vi "MecaDrivePoseEst2_ResetPosition.vi"(6 "Pose":T7={"TRANSLATION"={"X"=0.0, "Y"=0.0}, "ROTATION"={"VALUE"=0.0, "COS"=1.0, "SIN"=0.0}} {"ROTATION"."SIN" format="%13.4f"; "ROTATION"."COS" format="%13.4f"; "ROTATION"."VALUE" format="%13.4f"; "TRANSLATION"."Y" format="%14.3f"; "TRANSLATION"."X" format="%14.3f"}, 9 "Module Positions":T1 {"RearRight" format="%19.3f"; "RearLeft" format="%19.3f"; "FrontRight" format="%19.3f"; "FrontLeft" format="%19.3f"}, 10 "Gyro":T2={"VALUE"=0.0, "COS"=1.0, "SIN"=0.0} {"SIN" format="%13.4f"; "COS" format="%13.4f"; "VALUE" format="%13.4f"}, 11 "in MecaDrivePoseEst2":T3={"M_Vision_K"=[], "m_nominal_dT"=0.0, "m_PrevTime_Sec"=0.0, "Pose_Buffer"={"TimeStamps"=[], "DataArray"=[], "Min_TimeStamp"=0.0, "Max_TimeStamp"=0.0, "ItemCount"=0, "MaxBufferTime"=0.0}, "Meca_Drive_Odom"={"POSE"={"TRANSLATION"={"X"=0.0, "Y"=0.0}, "ROTATION"={"VALUE"=0.0, "COS"=1.0, "SIN"=0.0}}, "GyroOffset"={"VALUE"=0.0, "COS"=1.0, "SIN"=0.0}, "PreviousAngle"={"VALUE"=0.0, "COS"=1.0, "SIN"=0.0}, "Kinematics"={"FrontLeft"={"X"=0.0, "Y"=0.0}, "FrontRight"={"X"=0.0, "Y"=0.0}, "RearLeft"={"X"=0.0, "Y"=0.0}, "RearRight"={"X"=0.0, "Y"=0.0}, "InverseKinematics"=[[0.0, 1.0, -1.0, 0.0], [0.0, 1.0, 1.0, 0.0], [0.0, 1.0, 1.0, 0.0], [0.0, 1.0, -1.0, 0.0]], "ForwardKinematics"=[[0.0, 1.0, -1.0, 0.0], [0.0, 1.0, 1.0, 0.0], [0.0, 1.0, 1.0, 0.0], [0.0, 1.0, -1.0, 0.0]], "PrevCoR"={"X"=0.0, "Y"=0.0}}, "PreviousWheelPositions"={"FrontLeft"=0.0, "FrontRight"=0.0, "RearLeft"=0.0, "RearRight"=0.0, "P"=FALSE}}, "M_Q"=[[0.0], [0.0], [0.0]]} {"Meca_Drive_Odom"."PreviousWheelPositions"."RearRight" format="%19.3f"; "Meca_Drive_Odom"."PreviousWheelPositions"."RearLeft" format="%19.3f"; "Meca_Drive_Odom"."PreviousWheelPositions"."FrontRight" format="%19.3f"; "Meca_Drive_Odom"."PreviousWheelPositions"."FrontLeft" format="%19.3f"; "Meca_Drive_Odom"."Kinematics"."PrevCoR"."Y" format="%14.3f"; "Meca_Drive_Odom"."Kinematics"."PrevCoR"."X" format="%14.3f"; "Meca_Drive_Odom"."Kinematics"."RearRight"."Y" format="%14.3f"; "Meca_Drive_Odom"."Kinematics"."RearRight"."X" format="%14.3f"; "Meca_Drive_Odom"."Kinematics"."RearLeft"."Y" format="%14.3f"; "Meca_Drive_Odom"."Kinematics"."RearLeft"."X" format="%14.3f"; "Meca_Drive_Odom"."Kinematics"."FrontRight"."Y" format="%14.3f"; "Meca_Drive_Odom"."Kinematics"."FrontRight"."X" format="%14.3f"; "Meca_Drive_Odom"."Kinematics"."FrontLeft"."Y" format="%14.3f"; "Meca_Drive_Odom"."Kinematics"."FrontLeft"."X" format="%14.3f"; "Meca_Drive_Odom"."PreviousAngle"."SIN" format="%13.4f"; "Meca_Drive_Odom"."PreviousAngle"."COS" format="%13.4f"; "Meca_Drive_Odom"."PreviousAngle"."VALUE" format="%13.4f"; "Meca_Drive_Odom"."GyroOffset"."SIN" format="%13.4f"; "Meca_Drive_Odom"."GyroOffset"."COS" format="%13.4f"; "Meca_Drive_Odom"."GyroOffset"."VALUE" format="%13.4f"; "Meca_Drive_Odom"."POSE"."ROTATION"."SIN" format="%13.4f"; "Meca_Drive_Odom"."POSE"."ROTATION"."COS" format="%13.4f"; "Meca_Drive_Odom"."POSE"."ROTATION"."VALUE" format="%13.4f"; "Meca_Drive_Odom"."POSE"."TRANSLATION"."Y" format="%14.3f"; "Meca_Drive_Odom"."POSE"."TRANSLATION"."X" format="%14.3f"}) -> (3 "Out MecaDrivePoseEst2":T3={"M_Vision_K"=[], "m_nominal_dT"=0.0, "m_PrevTime_Sec"=0.0, "Pose_Buffer"={"TimeStamps"=[], "DataArray"=[], "Min_TimeStamp"=0.0, "Max_TimeStamp"=0.0, "ItemCount"=0, "MaxBufferTime"=0.0}, "Meca_Drive_Odom"={"POSE"={"TRANSLATION"={"X"=0.0, "Y"=0.0}, "ROTATION"={"VALUE"=0.0, "COS"=1.0, "SIN"=0.0}}, "GyroOffset"={"VALUE"=0.0, "COS"=1.0, "SIN"=0.0}, "PreviousAngle"={"VALUE"=0.0, "COS"=1.0, "SIN"=0.0}, "Kinematics"={"FrontLeft"={"X"=0.0, "Y"=0.0}, "FrontRight"={"X"=0.0, "Y"=0.0}, "RearLeft"={"X"=0.0, "Y"=0.0}, "RearRight"={"X"=0.0, "Y"=0.0}, "InverseKinematics"=[[0.0, 1.0, -1.0, 0.0], [0.0, 1.0, 1.0, 0.0], [0.0, 1.0, 1.0, 0.0], [0.0, 1.0, -1.0, 0.0]], "ForwardKinematics"=[[0.0, 1.0, -1.0, 0.0], [0.0, 1.0, 1.0, 0.0], [0.0, 1.0, 1.0, 0.0], [0.0, 1.0, -1.0, 0.0]], "PrevCoR"={"X"=0.0, "Y"=0.0}}, "PreviousWheelPositions"={"FrontLeft"=0.0, "FrontRight"=0.0, "RearLeft"=0.0, "RearRight"=0.0, "P"=FALSE}}, "M_Q"=[[0.0], [0.0], [0.0]]} {"Meca_Drive_Odom"."PreviousWheelPositions"."RearRight" format="%19.3f"; "Meca_Drive_Odom"."PreviousWheelPositions"."RearLeft" format="%19.3f"; "Meca_Drive_Odom"."PreviousWheelPositions"."FrontRight" format="%19.3f"; "Meca_Drive_Odom"."PreviousWheelPositions"."FrontLeft" format="%19.3f"; "Meca_Drive_Odom"."Kinematics"."PrevCoR"."Y" format="%14.3f"; "Meca_Drive_Odom"."Kinematics"."PrevCoR"."X" format="%14.3f"; "Meca_Drive_Odom"."Kinematics"."RearRight"."Y" format="%14.3f"; "Meca_Drive_Odom"."Kinematics"."RearRight"."X" format="%14.3f"; "Meca_Drive_Odom"."Kinematics"."RearLeft"."Y" format="%14.3f"; "Meca_Drive_Odom"."Kinematics"."RearLeft"."X" format="%14.3f"; "Meca_Drive_Odom"."Kinematics"."FrontRight"."Y" format="%14.3f"; "Meca_Drive_Odom"."Kinematics"."FrontRight"."X" format="%14.3f"; "Meca_Drive_Odom"."Kinematics"."FrontLeft"."Y" format="%14.3f"; "Meca_Drive_Odom"."Kinematics"."FrontLeft"."X" format="%14.3f"; "Meca_Drive_Odom"."PreviousAngle"."SIN" format="%13.4f"; "Meca_Drive_Odom"."PreviousAngle"."COS" format="%13.4f"; "Meca_Drive_Odom"."PreviousAngle"."VALUE" format="%13.4f"; "Meca_Drive_Odom"."GyroOffset"."SIN" format="%13.4f"; "Meca_Drive_Odom"."GyroOffset"."COS" format="%13.4f"; "Meca_Drive_Odom"."GyroOffset"."VALUE" format="%13.4f"; "Meca_Drive_Odom"."POSE"."ROTATION"."SIN" format="%13.4f"; "Meca_Drive_Odom"."POSE"."ROTATION"."COS" format="%13.4f"; "Meca_Drive_Odom"."POSE"."ROTATION"."VALUE" format="%13.4f"; "Meca_Drive_Odom"."POSE"."TRANSLATION"."Y" format="%14.3f"; "Meca_Drive_Odom"."POSE"."TRANSLATION"."X" format="%14.3f"})   [LabVIEW 2019, in "Trajectory_Library.lvlib"]
doc: "Resets the robot's position on the field.\n \nThe gyroscope angle does not need to be reset here on the user's robot code. The library automatically takes care of offsetting the gyro angle.\n \nInputs:\n - inSwerveDrvPoseEst2 -- SwerveDrvPoseEst2 -- Data cluster\n - gyroAngle -- Rotation2d -- The angle reported by the gyroscope.\n - ModulePositions -- ModulePositions -- The current module positions.\n - poseMeters -- Pose2d -- The position on the field that your robot is at.\n\nOutputs:\n - outSwerveDrvPoseEst2 -- SwerveDrvPoseEst2 -- Updated data cluster"
uses:
  Trajectory_Library.lvlib
  TypeDef/MECA_DRIVE_POSE_EST2.ctl
  <vilib>/Analysis/Matrix/Datatypes/RealMatrix.ctl
  TypeDef/TIME_INTERPOLATABLE_VARIANT.ctl
  TypeDef/MECA_DRIVE_ODOMETRY.ctl
  TypeDef/POSE2D.ctl
  TypeDef/TRANSLATION2D.ctl
  TypeDef/ROTATION2D.ctl
  TypeDef/MECA_DRIVE_KINEMATICS.ctl
  TypeDef/MECA_WHEEL_POSITIONS.ctl
  <vilib>/Analysis/Matrix/NI_Matrix.lvlib
panel:
  # "<3, 1>"
  # "<3, 3>"
  # "<3, 1>"
  # "<3, 3>"
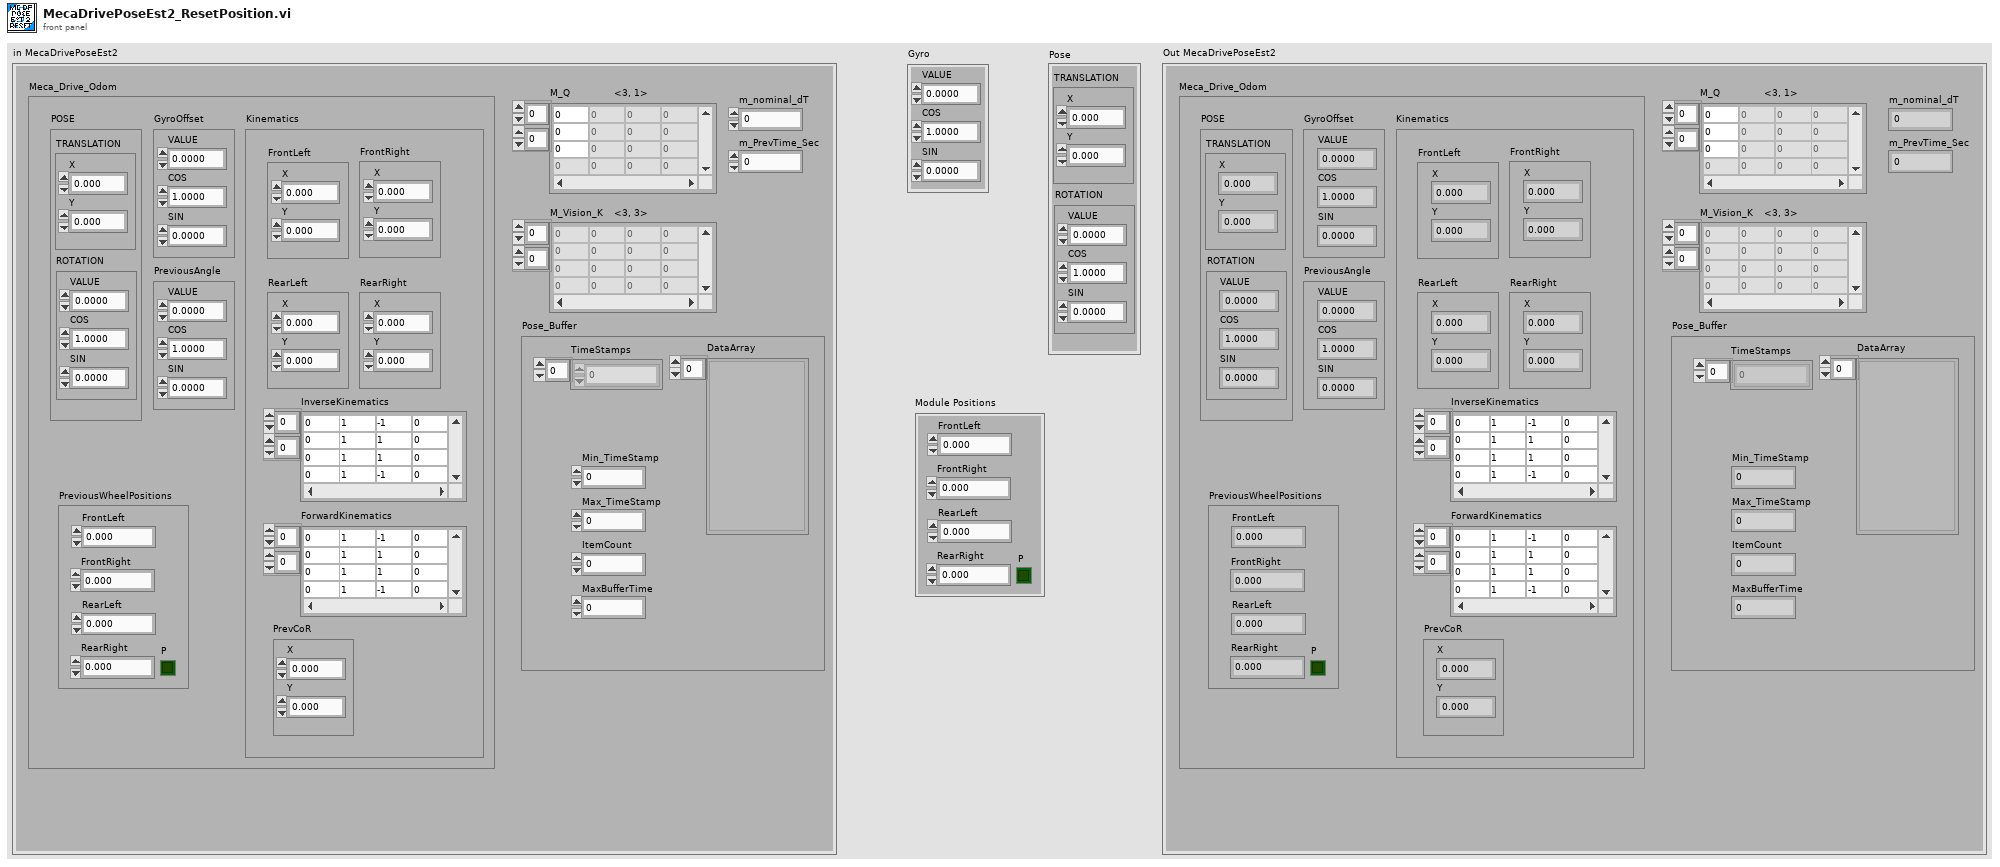
[diagram p1: front panel]
types:
  T1 = typedef "Trajectory_Library.lvlib/MECA_WHEEL_POSITIONS.ctl" = cluster{"FrontLeft":dbl, "FrontRight":dbl, "RearLeft":dbl, "RearRight":dbl, "P":bool}
  T2 = typedef "Trajectory_Library.lvlib/ROTATION2D.ctl" = cluster{"VALUE":dbl, "COS":dbl, "SIN":dbl}
  T3 = typedef "Trajectory_Library.lvlib/MECA_DRIVE_POSE_EST2.ctl" = cluster{"M_Vision_K":T4, "m_nominal_dT":dbl, "m_PrevTime_Sec":dbl, "Pose_Buffer":T5, "Meca_Drive_Odom":T6, "M_Q":T4}
  T4 = typedef "NI_Matrix.lvlib/RealMatrix.ctl" = dbl[][]
  T5 = typedef "Trajectory_Library.lvlib/TIME_INTERPOLATABLE_VARIANT.ctl" = cluster{"TimeStamps":dbl[], "DataArray":variant[], "Min_TimeStamp":dbl, "Max_TimeStamp":dbl, "ItemCount":i32, "MaxBufferTime":dbl}
  T6 = typedef "Trajectory_Library.lvlib/MECA_DRIVE_ODOMETRY.ctl" = cluster{"POSE":T7, "GyroOffset":T2, "PreviousAngle":T2, "Kinematics":T9, "PreviousWheelPositions":T1}
  T7 = typedef "Trajectory_Library.lvlib/POSE2D.ctl" = cluster{"TRANSLATION":T8, "ROTATION":T2}
  T8 = typedef "Trajectory_Library.lvlib/TRANSLATION2D.ctl" = cluster{"X":dbl, "Y":dbl}
  T9 = typedef "Trajectory_Library.lvlib/MECA_DRIVE_KINEMATICS.ctl" = cluster{"FrontLeft":T8, "FrontRight":T8, "RearLeft":T8, "RearRight":T8, "InverseKinematics":T4, "ForwardKinematics":T4, "PrevCoR":T8}
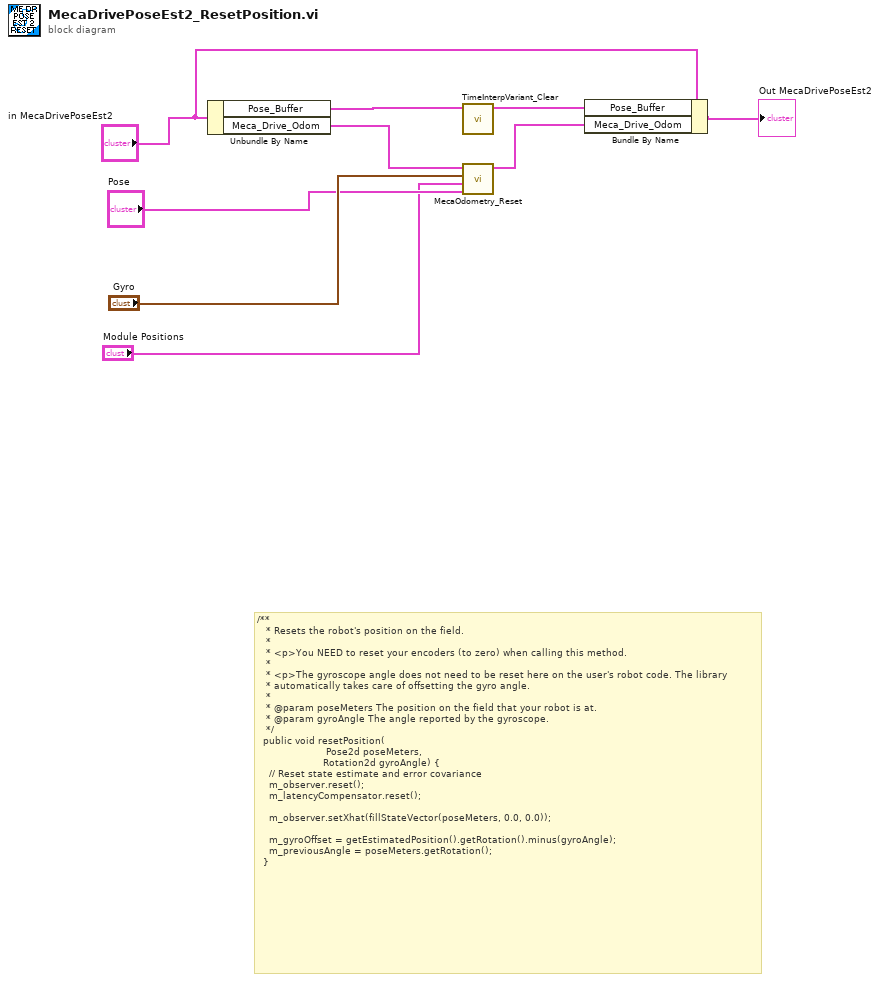
[diagram p0: block diagram]
diagram:
  # "/**\n   * Resets the robot's position on the field.\n   *\n   * <p>You NEED to reset your encoders (to zero) when calling this method.\n   *\n   * <p>The gyroscope angle does not need to be reset here on the user's robot code. The library\n   * automatically takes care of offsetting the gyro angle.\n   *\n   * @param poseMeters The position on the field that your robot is at.\n   * @param gyroAngle The angle reported by the gyroscope.\n   */\n  public void resetPosition(\n                       Pose2d poseMeters, \n                      Rotation2d gyroAngle) {\n    // Reset state estimate and error covariance\n    m_observer.reset();\n    m_latencyCompensator.reset();\n\n    m_observer.setXhat(fillStateVector(poseMeters, 0.0, 0.0));\n\n    m_gyroOffset = getEstimatedPosition().getRotation().minus(gyroAngle);\n    m_previousAngle = poseMeters.getRotation();\n  }"
  n1 = Unbundle By Name("in MecaDrivePoseEst2") -> ("Pose_Buffer"=w8:T5, "Meca_Drive_Odom"=w5:T6)
  n2 = call "TimeInterpVariant_Clear.vi"("in TimeInterpVariant"=w8) -> ("out TimeInterpVariant"=w7:T5)  [unwired: 10 in]
  n3 = call "MecaOdometry_Reset.vi"("POSE"="Pose", "WheelPositions"="Module Positions", "GyroOffset"="Gyro", "in MECA_DRIVE_ODOMETRY"=w5) -> ("out MECA_DRIVE_ODOMETRY"=w4:T6)  [unwired: 7 in]
  n4 = Bundle By Name(cluster="in MecaDrivePoseEst2", "Pose_Buffer"=w7, "Meca_Drive_Odom"=w4) -> (→"Out MecaDrivePoseEst2":T3)
